vi "ESC_Open serial port.vi"(10 "timeout (ms)":u32=10000, 11 "VISA resource name":refnum<visa-resource-name>) -> (0 "Error out":errorcluster, 3 "VISA resource name out":refnum<visa-resource-name>)   [LabVIEW 2018]
uses:
  <vilib>/Instr/_visa.llb/VISA Open Access Mode.ctl
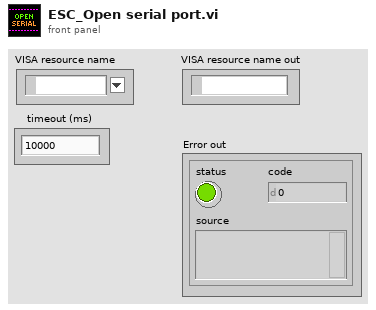
[diagram p1: front panel]
types:
  T1 = typedef "VISA Open Access Mode.ctl" = u32
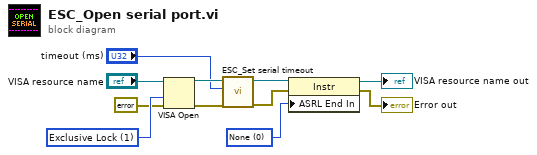
[diagram p0: block diagram]
diagram:
  w8 = u16 0 items=["None", "Last Bit", "TermChar"] ("Serial Settings:End Mode for Reads")
  w11 = T1 1 items=["VISA Defaults"=0, "Exclusive Lock"=1, "Load Configured Settings"=4] ("Access Mode")
  n1 = VISA Open(access mode=w11, error in (no error)=errorcluster {"status"=FALSE, "code"=0, "source"=""}, VISA resource name="VISA resource name") -> (VISA resource name=w4:refnum<visa-resource-name>, error out=w5:errorcluster)  [unwired: 2 in]
  n2 = call "ESC_Set serial timeout.vi"("Error In"=w5, "timeout (ms)"="timeout (ms)", "VISA resource name"=w4) -> ("Error Out"=w2:errorcluster, "VISA resource name out"=w3:refnum<visa-resource-name>)  [unwired: 7 in]
  n3 = property class="Instr"(reference=w3, error in=w2, "ASRL End In"=w8) -> (reference out=→"VISA resource name out":refnum<visa-resource-name>, error out=→"Error out":errorcluster)
